vi "Functional data-Reshape MSCN data to 1D array.vi"(11 "Single miniscan single trial data":u32[][](array[numeric])=[[1, 2, 3, 4, 5], [6, 7, 8, 9, 10], [11, 12, 13, 14, 15]]) -> (3 "Reshaped array (1D)":u32[](array[numeric]))   [LabVIEW 2020]
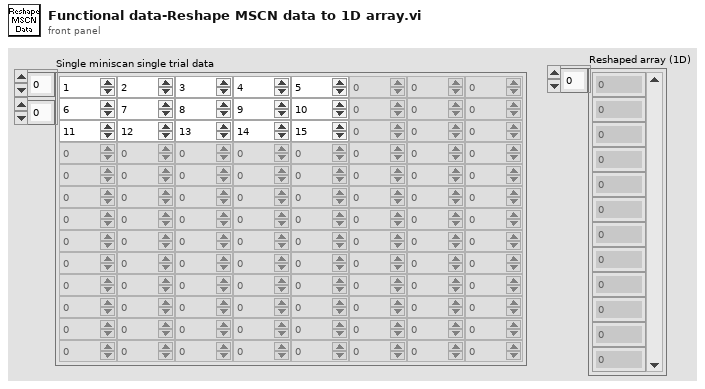
[diagram p1: front panel]
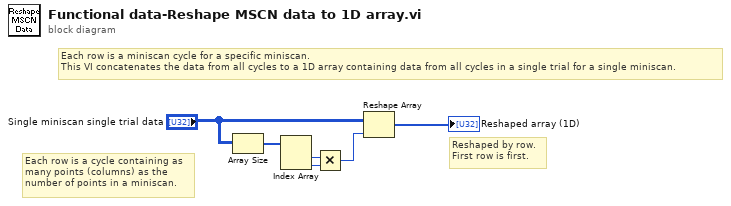
[diagram p0: block diagram]
diagram:
  # "Each row is a cycle containing as many points (columns) as the number of points in a miniscan."
  # "Each row is a miniscan cycle for a specific miniscan.\nThis VI concatenates the data from all cycles to a 1D array containing data from all cycles in a single trial for a single miniscan."
  # "Reshaped by row.\nFirst row is first."
  n1 = Array Size(array="Single miniscan single trial data") -> (size(s)=w4:i32[])
  n2 = Index Array(array=w4) -> (element #1=w3:i32, element #2=w2:i32)  [unwired: 2 in]
  n3 = Multiply(x=w3, y=w2) -> (x*y=w1:i32)
  n4 = Reshape Array "Reshape Array"("Single miniscan single trial data", w1) -> (→"Reshaped array (1D)":u32[])
